vi "CalcSSD.vi"   [LabVIEW 2014]
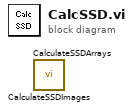
[diagram p0: block diagram]
diagram:
  n1 = call "CalculateSSDImages.vi"() -> ()  [unwired: 11 in, 1 out]
  n2 = call "CalculateSSDArrays.vi"() -> ()  [unwired: 11 in, 1 out]
